vi "init_panel.vi"(0 "Vali File Loaded?":refnum<vi>, 1 "Starttime":refnum<vi>, 2 "Endtime":refnum<vi>, 3 "# Iterations":refnum<vi>, 5 "Spec File Loaded?":refnum<vi>, 7 "Run Button":refnum<vi>, 9 "Sim File Loaded?":refnum<vi>, 11 "Parameters Tree":refnum<vi>) -> ()   [LabVIEW 2019]
uses:
  lib/libSpecValiReader.so
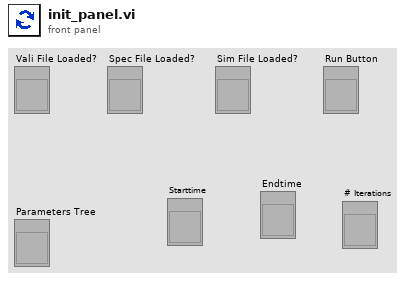
[diagram p1: front panel]
types:
  T1 = enum8{"Enabled", "Disabled", "Disabled and Grayed Out"}
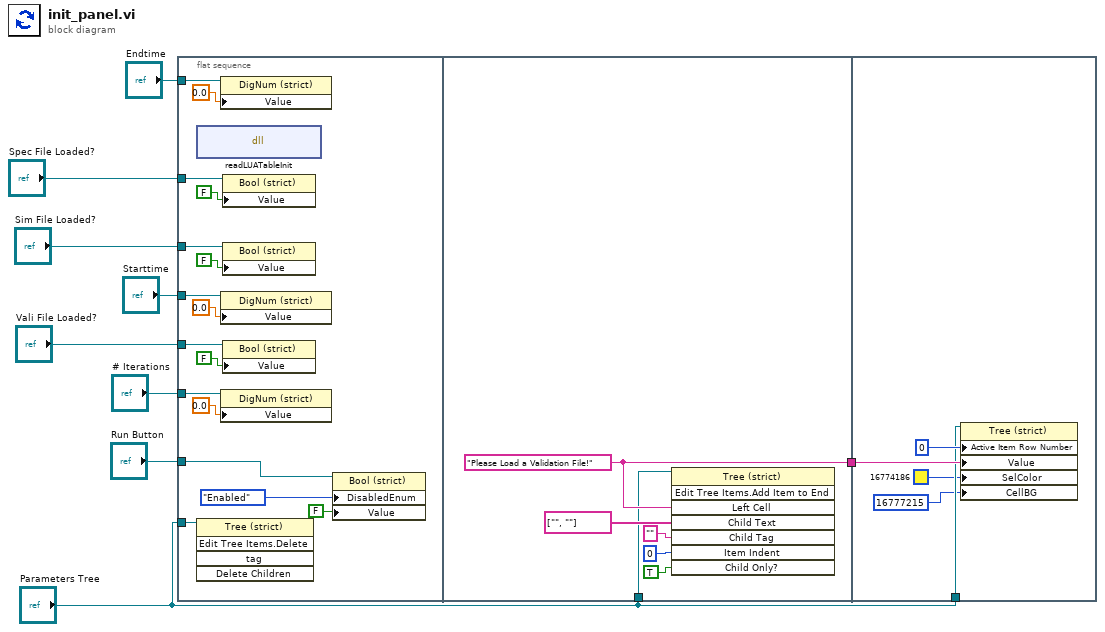
[diagram p0: block diagram]
diagram:
  n1 = flat-sequence {
    tunnel: "Vali File Loaded?" -> [w24]
    tunnel: "Parameters Tree" -> [w23]
    tunnel: "Spec File Loaded?" -> [w22]
    tunnel: "Sim File Loaded?" -> [w19]
    tunnel: "# Iterations" -> [w18]
    tunnel: "Starttime" -> [w16]
    tunnel: "Endtime" -> [w15]
    tunnel: "Run Button" -> [w12]
    tunnel: [w28] -> w9
    tunnel: "Parameters Tree" -> [w26]
    tunnel: w9 -> [w35]
    tunnel: "Parameters Tree" -> [w34]
    frame #0 {
      n2 = dll-call lib="home/paul/Schreibtisch/Biogas_plant_setup/lib/libSpecValiReader.so" fn="readLUATableInit"() -> ()  [unwired: 4 in, 2 out]
      n3 = invoke on="Invoke Node" class="Tree (strict)" method="Edit Tree Items.Delete"(reference=w23) -> ()  [unwired: 4 in, 5 out]
      n4 = property class="DigNum (strict)"(reference=w15, "Value"=0.0) -> ()  [unwired: 1 in, 2 out]
      n5 = property class="DigNum (strict)"(reference=w16, "Value"=0.0) -> ()  [unwired: 1 in, 2 out]
      n6 = property class="DigNum (strict)"(reference=w18, "Value"=0.0) -> ()  [unwired: 1 in, 2 out]
      n7 = property class="Bool (strict)"(reference=w22, "Value"=FALSE) -> ()  [unwired: 1 in, 2 out]
      n8 = property class="Bool (strict)"(reference=w19, "Value"=FALSE) -> ()  [unwired: 1 in, 2 out]
      n9 = property class="Bool (strict)"(reference=w24, "Value"=FALSE ("Vali File Loaded")) -> ()  [unwired: 1 in, 2 out]
      n10 = property class="Bool (strict)"(reference=w12, "DisabledEnum"=T1."Enabled" ("Disabled"), "Value"=FALSE ("Blinking")) -> ()  [unwired: 1 in, 2 out]
    }
    frame #1 {
      w28 = "Please Load a Validation File!" ("Parent Tag")
      n11 = invoke on="Invoke Node" class="Tree (strict)" method="Edit Tree Items.Add Item to End"(reference=w26, "Left Cell"=w28, "Child Text"=string[] ["", ""], "Child Tag"="", "Item Indent"=0 ("New Item Indentation"), "Child Only?"=TRUE) -> ()  [unwired: 2 in, 8 out]
    }
    frame #2 {
      n12 = property on="Property Node" class="Tree (strict)"(reference=w34, "Active Item Row Number"=0 ("Active Item:Row Number"), "Value"=w35, "SelColor"=u32 16774186, "CellBG"=u32 16777215 ("Active Cell:Background Color")) -> ()  [unwired: 1 in, 2 out]
    }
  }
